vi "Write Module.vi"(5 "Channel Type":T5, 7 "R/W Case":T4, 8 "error in (no error)":errorcluster, 9 "Input FIFO buffer in":dbl[](array[numeric]), 10 "Input Data in":T1 {"BD Refs"."Data Reference" format="%.0x"}, 11 "IOV ref in":T6) -> (0 "error out":errorcluster, 1 "Input FIFO buffer out":dbl[](array[numeric]), 2 "Input Data out":T1 {"BD Refs"."Data Reference" format="%.0x"}, 3 "IOV ref out":T6)   [LabVIEW 2011, in "Scan Engine Custom Device.lvlib"]
uses:
  Scan Engine Custom Device.lvlib
  Type Defs/Open Module IOVs.ctl
  Modules.lvlibp/RSI Module/Channel Type.ctl
  Type Defs/RW Case.ctl
  Type Defs/Input Data.ctl
  <vilib>/NI Veristand/Custom Device API/Block Data Reference.ctl
  <vilib>/NI Veristand/Custom Device API/Data Reference.ctl
  <vilib>/NI Veristand/Custom Device API/Global Data Refs.vi
  <vilib>/NI Veristand/Custom Device API/Custom Device API.lvlib
  Modules.lvlibp/RSI Module/RSI Module.lvclass
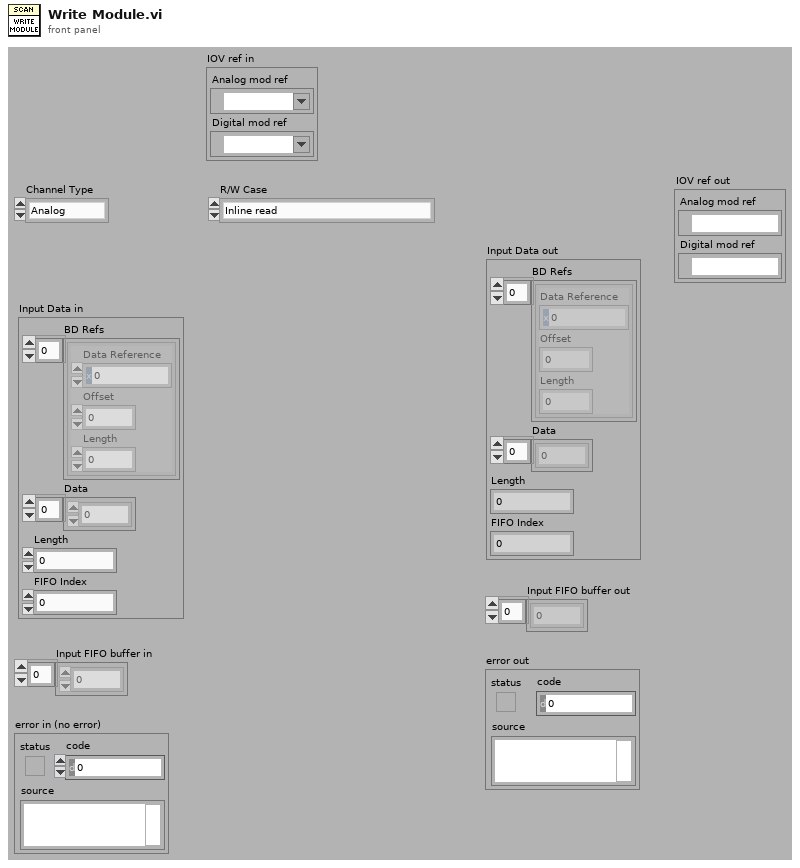
[diagram p1: front panel]
types:
  T1 = typedef "Scan Engine Custom Device.lvlib/Input Data.ctl" = cluster{"BD Refs":T2[], "Data":dbl[], "Length":i32, "FIFO Index":i32}
  T2 = typedef "Custom Device API.lvlib/Block Data Reference.ctl" = cluster{"Data Reference":T3, "Offset":i32, "Length":i32}
  T3 = typedef "Custom Device API.lvlib/Data Reference.ctl" = i32
  T4 = typedef "Scan Engine Custom Device.lvlib/RW Case.ctl" = enum16{"Inline read", "Inline write", "Async - Inline loop read", "Async - Inline loop write", "Async loop (read/write)"}
  T5 = typedef "Modules.lvlibp/RSI Module.lvclass/Channel Type.ctl" = enum16{"Analog", "Digital"}
  T6 = typedef "Scan Engine Custom Device.lvlib/Open Module IOVs.ctl" = cluster{"Analog mod ref":refnum<k21>, "Digital mod ref":refnum<k21>}
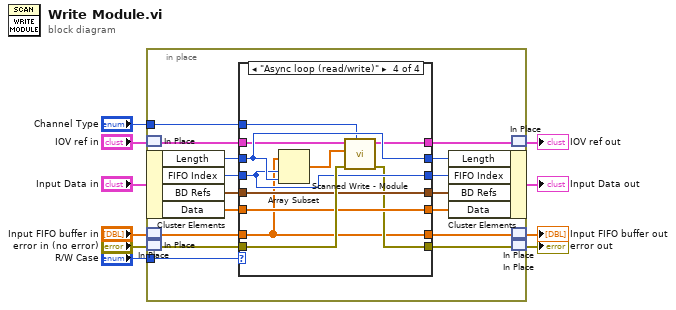
[diagram p0: block diagram]
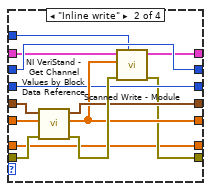
[diagram p3: hidden frame]
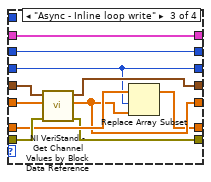
[diagram p4: hidden frame]
diagram:
  n1 = in-place {
    in-place-border: "R/W Case" -> [w26]
    in-place-border: "Channel Type" -> [w25]
    n2 = in-place-match #1("IOV ref in") -> (w14:T6)
    n3 = in-place-cluster #2("Input Data in") -> ("Length"=w17:i32, "FIFO Index"=w20:i32, "BD Refs"=w23:T2[], "Data"=w24:dbl[])
    n4 = in-place-match #3("Input FIFO buffer in") -> (w16:dbl[])
    n5 = in-place-match #4("error in (no error)") -> (w12:errorcluster)
    n6 = case shown="\"Async loop (read/write)\"" w26 {
      tunnel: w12 -> [w27 w46 w57 w68]
      tunnel: w16 -> [w28 w34 w54 w58]
      tunnel: w17 -> [w31 w40 w51 w64]
      tunnel: w20 -> [w32 w39 w50 w63]
      tunnel: w23 -> [w30 w45 w56 w66]
      tunnel: w24 -> [w29 w44 w55 w67]
      tunnel: [w29 w41 w52 w67] -> w21
      tunnel: [w30 w42 w53 w66] -> w22
      tunnel: [w31 w40 w51 w64] -> w18
      tunnel: [w32 w39 w50 w63] -> w19
      tunnel: [w33 w38 w49 w62] -> w13
      tunnel: w14 -> [w33 w37 w49 w61]
      tunnel: w25 -> [_ w36 _ w60]
      tunnel: [w27 w35 w48 w59] -> w11
      tunnel: [w28 w34 w47 w58] -> w15
      frame Default {
      }
      frame "Inline write" {
        n7 = call <vilib>:"NI VeriStand - Get Channel Values by Block Data Reference.vi"("error in (no error)"=w46, "Values Array in"=w44, "Block Data Ref"=w45) -> ("error out"=w43:errorcluster, "Values Array out"=w41:dbl[], "Block Data Ref dup"=w42:T2[])  [unwired: 6 in]
        n8 = call "Scanned Write - Module.vi"("Channel Type"=w36, "error in (no error)"=w43, "data in"=w41, "IOV ref in"=w37) -> ("error out"=w35:errorcluster, "IOV ref out"=w38:T6)  [unwired: 5 in]
      }
      frame "Async - Inline loop write" {
        n9 = call <vilib>:"NI VeriStand - Get Channel Values by Block Data Reference.vi"("error in (no error)"=w57, "Values Array in"=w55, "Block Data Ref"=w56) -> ("error out"=w48:errorcluster, "Values Array out"=w52:dbl[], "Block Data Ref dup"=w53:T2[])  [unwired: 6 in]
        n10 = Replace Array Subset(array=w54, new element=w52, index=w50) -> (w47:dbl[])
      }
      frame "Async loop (read/write)" {
        n11 = Array Subset(array=w58, index=w63, length=w64) -> (w65:dbl[])
        n12 = call "Scanned Write - Module.vi"("Channel Type"=w60, "error in (no error)"=w68, "data in"=w65, "IOV ref in"=w61) -> ("error out"=w59:errorcluster, "IOV ref out"=w62:T6)  [unwired: 5 in]
      }
    }
    n13 = in-place-cluster #2("Length"=w18, "FIFO Index"=w19, "BD Refs"=w22, "Data"=w21) -> (→"Input Data out":T1)
    n14 = in-place-match #1(w13) -> (→"IOV ref out":T6)
    n15 = in-place-match #3(w15) -> (→"Input FIFO buffer out":dbl[])
    n16 = in-place-match #4(w11) -> (→"error out":errorcluster)
  }
